vi "ExtractScanFrame.vi"(6 "Header":T1, 10 "Scan Frame":i32, 11 "Scan Plane Data":dbl[][][](array[numeric])) -> (3 "Scan Frame Data":dbl[][](array[numeric]))   [LabVIEW 2011]
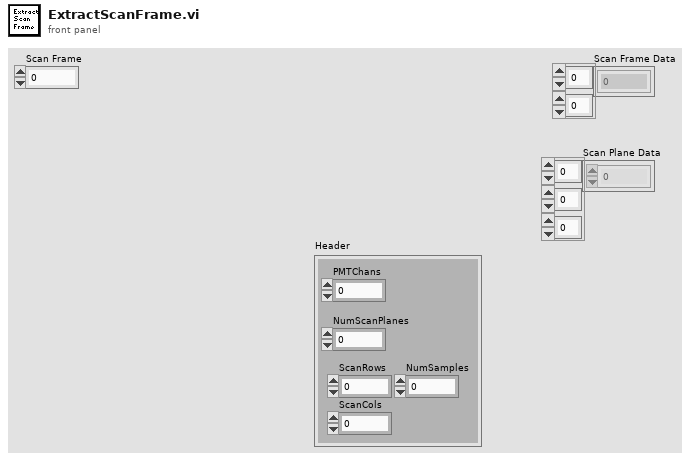
[diagram p1: front panel]
types:
  T1 = cluster{"PMTChans":i32, "NumScanPlanes":i32, "ScanRows":i32, "ScanCols":i32, "NumSamples":i32}
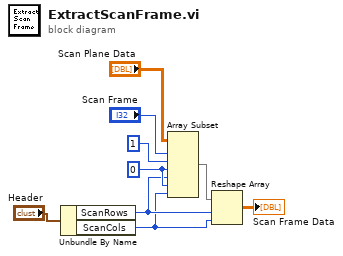
[diagram p0: block diagram]
diagram:
  w7 = 0 ("index")
  n1 = Unbundle By Name("Header") -> ("ScanRows"=w3:i32, "ScanCols"=w2:i32)
  n2 = Array Subset(array="Scan Plane Data", index (dim 0)="Scan Frame", length (dim 0)=1 ("length"), index (dim 1)=w7, length (dim 1)=w3, index (dim 2)=w7, length (dim 2)=w2) -> (w9:dbl[][][])
  n3 = Reshape Array(w9, w3, w2) -> (→"Scan Frame Data":dbl[][])
